vi "set_FPGA_ref.vi"(8 "error in":errorcluster, 11 "FPGA Reference":T1) -> (0 "error out":errorcluster)   [LabVIEW 2010, in "FPGAWrapperRK110909Throughput.lvclass"]
uses:
  FPGAWrapperRK110909Throughput.lvclass
  FPGA_reference.ctl
  class_data.vi
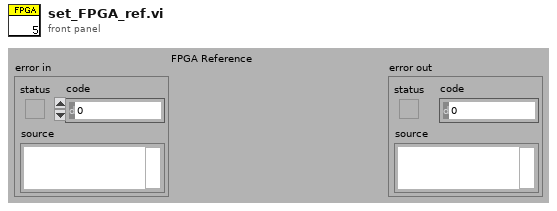
[diagram p1: front panel]
types:
  T1 = typedef "FPGAWrapperRK110909Throughput.lvclass/FPGA_reference.ctl" = refnum<k20>
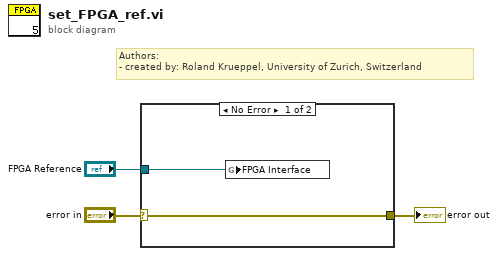
[diagram p0: block diagram]
diagram:
  # "Authors: \n- created by: Roland Krueppel, University of Zurich, Switzerland"
  n1 = case shown="No Error" "error in" {
    selector: "error in" -> [w5 w6]
    tunnel: [w5 w6] -> w1
    tunnel: "FPGA Reference" -> [w4 _]
    frame No Error {
      n2 = global write "class_data.vi" "FPGA Interface"(w4) -> ()
    }
    frame Error {
    }
  }
  "error out" <- w1
